vi "Save_Array_Data_to_File.vi"(4 "Raw Stiring?":bool, 5 "Raw String":string, 6 "Array format(%.5f)":string="%.5f", 7 "delimiter (comma)":string=",", 8 "error in":errorcluster, 9 "Header Array":string[](array[string]), 10 "Array":dbl[][](array[numeric]), 11 "file path (use dialog)":path) -> (0 "error out":errorcluster)   [LabVIEW 2015]
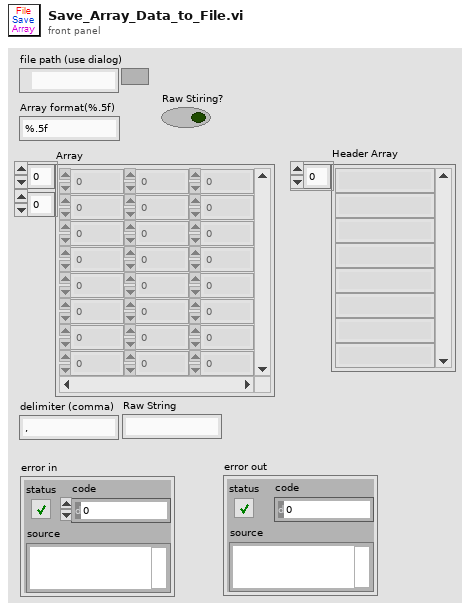
[diagram p1: front panel]
types:
  T1 = enum16{"open", "replace", "create", "open or create", "replace or create", "replace or create with confirmation"}
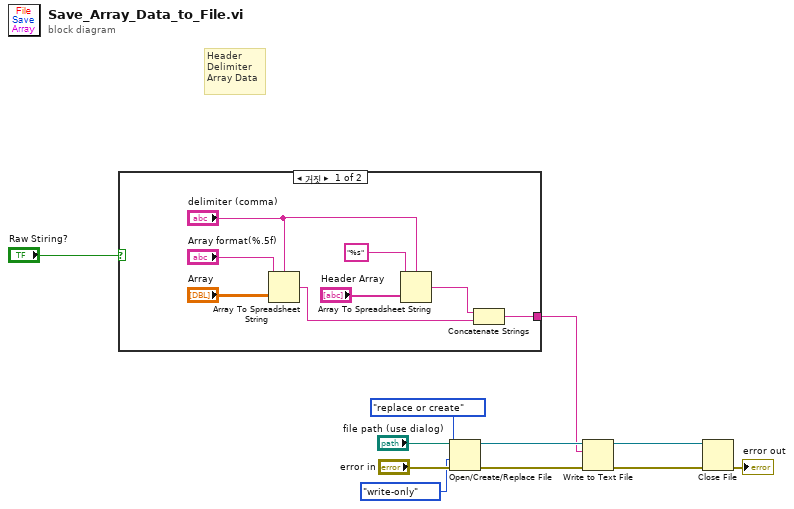
[diagram p0: block diagram]
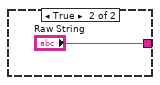
[diagram p2: hidden frame]
diagram:
  # "Header\nDelimiter\nArray Data"
  n1 = case shown="거짓" "Raw Stiring?" {
    tunnel: [w12 "Raw String"] -> w2
    frame False {
      n2 = Array To Spreadsheet String(delimiter (Tab)="delimiter (comma)", array="Array", 3:"Array format(%.5f)") -> (spreadsheet string=w13:string)
      n3 = Array To Spreadsheet String(delimiter (Tab)="delimiter (comma)", array="Header Array", 3:"%s" ("format string")) -> (spreadsheet string=w14:string)
      n4 = Concatenate Strings(w14, w13) -> (w12:string)
    }
    frame True {
    }
  }
  n5 = Open/Create/Replace File(file path (use dialog)="file path (use dialog)", error in="error in", operation (0:open)=T1."replace or create", access (0:read/write)=enum16{"read/write", "read-only", "write-only"}."write-only") -> (refnum out=w11:refnum<file>, error out=w10:errorcluster)  [unwired: 2 in, 1 out]
  n6 = Write to Text File(file (use dialog)=w11, text=w2, error in=w10) -> (refnum out=w9:refnum<file>, error out=w8:errorcluster)  [unwired: 1 in, 1 out]
  n7 = Close File(refnum=w9, error in=w8) -> (error out=→"error out":errorcluster)  [unwired: 1 out]
